vi "AsyncEngine.vi"(8 "Error In":errorcluster, 11 "AsyncDVR":refnum<data-value>) -> (0 "Error Out":errorcluster)   [LabVIEW 2019, in "MicronGRPCClient.lvclass"]
uses:
  MicronGRPCClient.lvclass
  Typedefs/AsyncCluster.ctl
  <vilib>/SLL Toolkit/SLL Queued State Machine/Queue Driver/Typedefs/Queue Type.ctl
  <vilib>/gRPC/LabVIEW gRPC Library/Shared/grpcId.ctl
  <vilib>/Utility/error.llb/DialogType.ctl
  <vilib>/SLL Toolkit/SLL Queued State Machine/Queue Driver/Enqueue an Item to Queue.vi
  <vilib>/SLL Toolkit/SLL Queued State Machine/Queue Driver/Dequeue Queue.vi
  <vilib>/SLL Toolkit/SLL Queued State Machine/Queue Driver/Enqueue N Items.vi
  <vilib>/SLL Toolkit/SLL Queued State Machine/Queue Driver/Flush Queue.vi
  <vilib>/SLL Toolkit/SLL Queued State Machine/Queue Driver/Release Queue.vi
  <vilib>/SLL Toolkit/SLL Queued State Machine/SLL QSM.lvlib
  <vilib>/gRPC/LabVIEW gRPC Library/grpc-lvsupport-release.lvlib
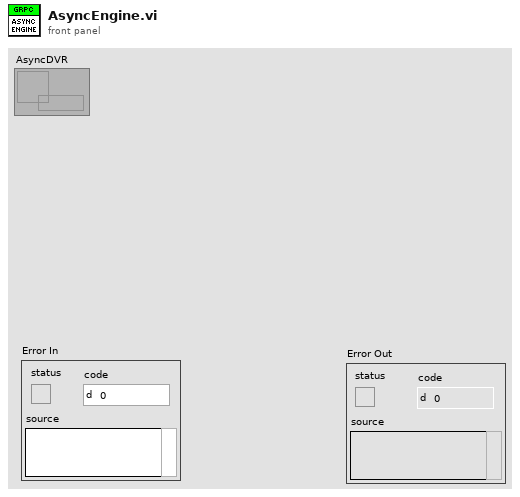
[diagram p1: front panel]
types:
  T1 = typedef "grpc-lvsupport-release.lvlib/grpcId.ctl" = u64
  T2 = cluster{"Flags":cluster{"Source Code?":bool}, "gRPC":cluster{"gRPC ID":T1, "PackageName":string, "ServiceName":string, "Simulate?":bool}}
  T3 = typedef "MicronGRPCClient.lvclass/AsyncCluster.ctl" = cluster{"QueueRef":refnum<queue>, "PackageName":string, "ServiceName":string, "gRPC ID":T1, "Simulate?":bool}
  T4 = typedef "DialogType.ctl" = u16
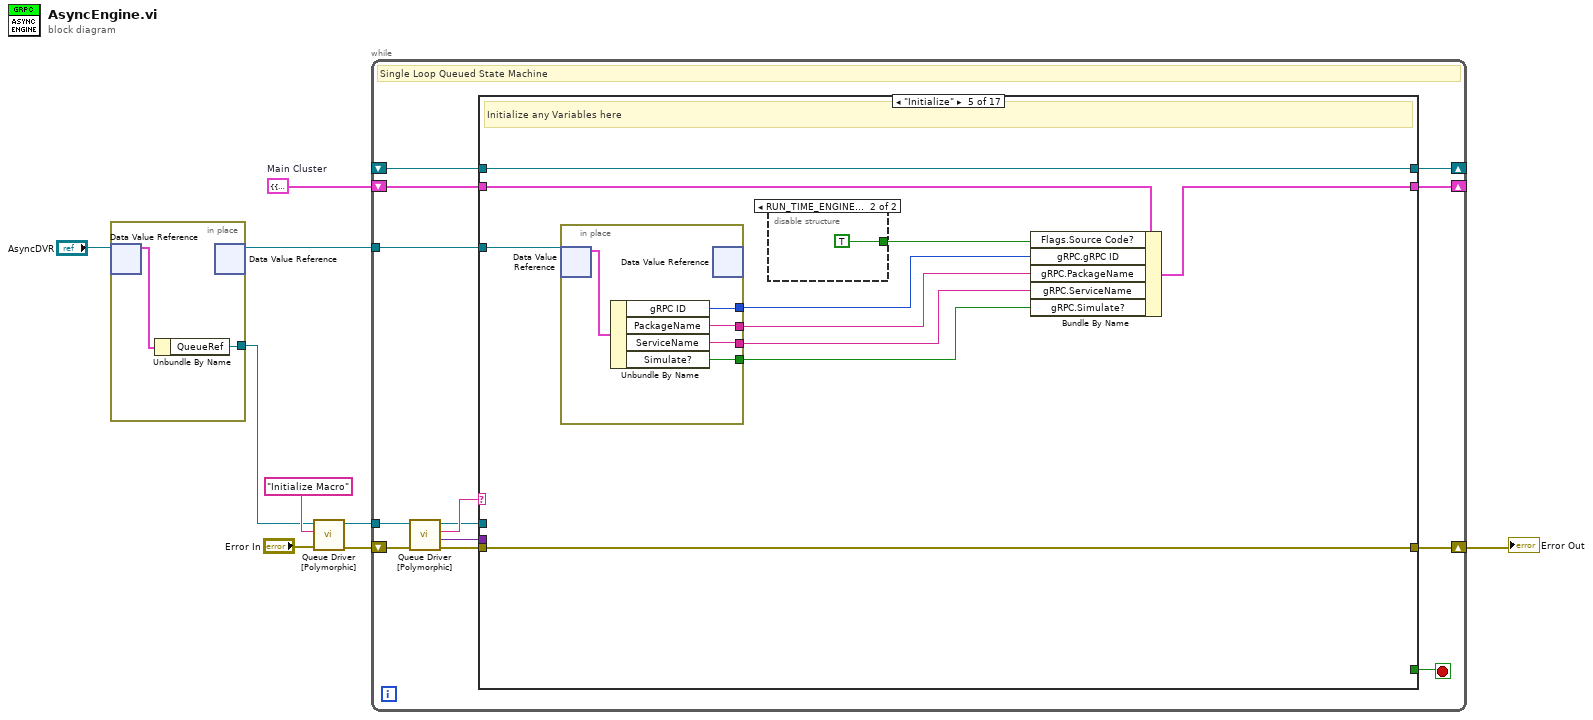
[diagram p0: block diagram]
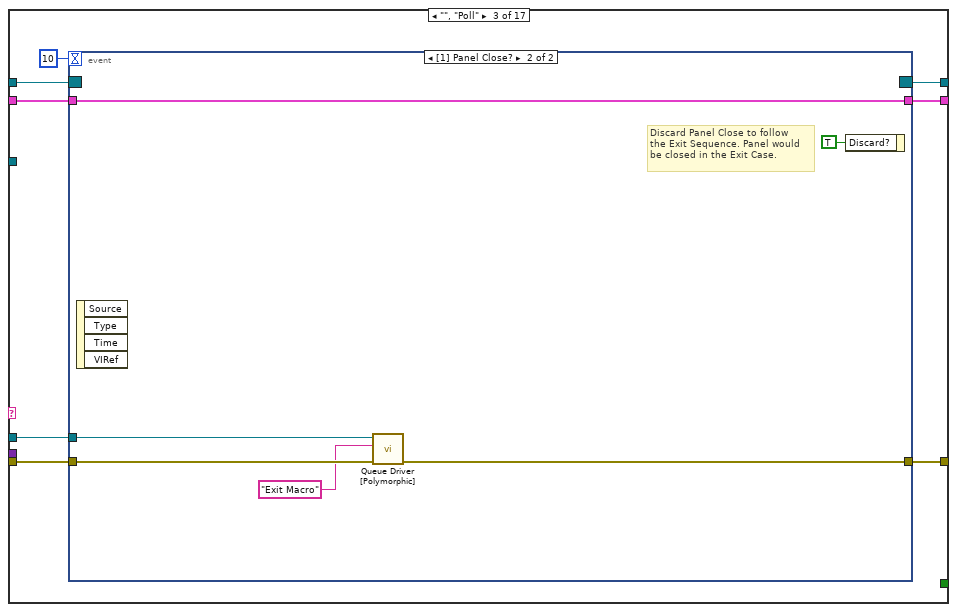
[diagram p4: hidden frame]
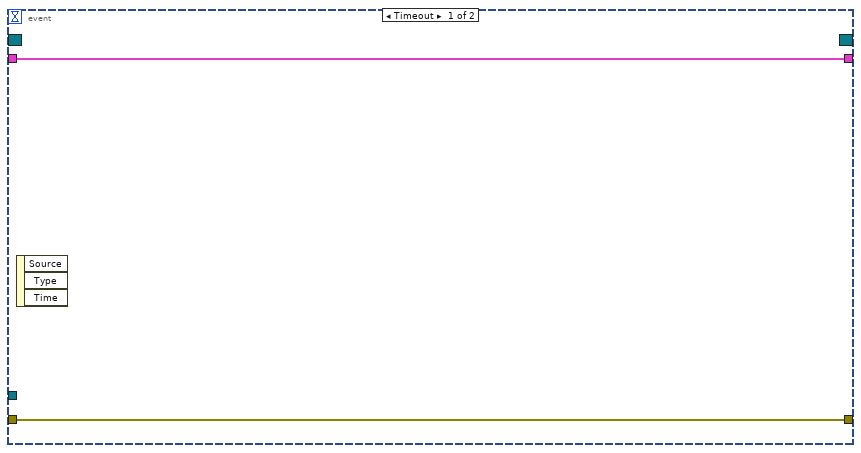
[diagram p5: hidden frame]
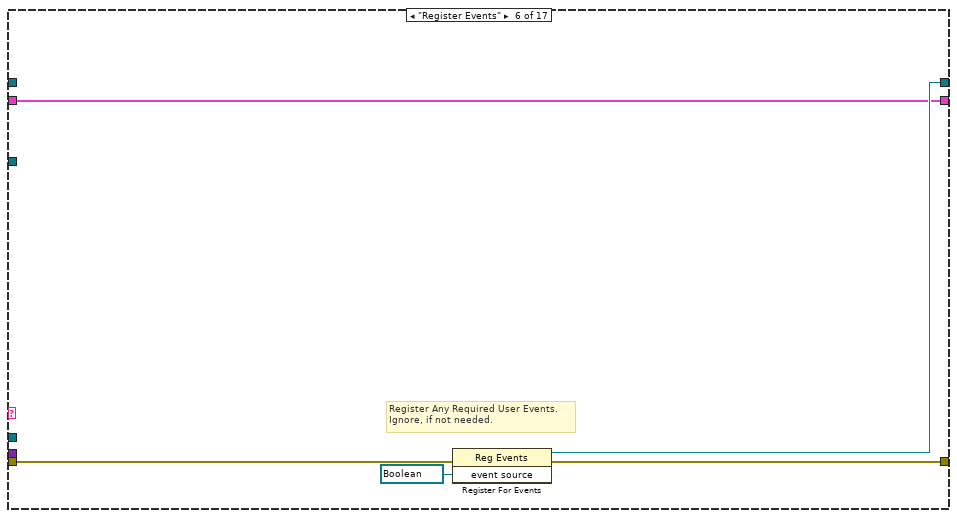
[diagram p8: hidden frame]
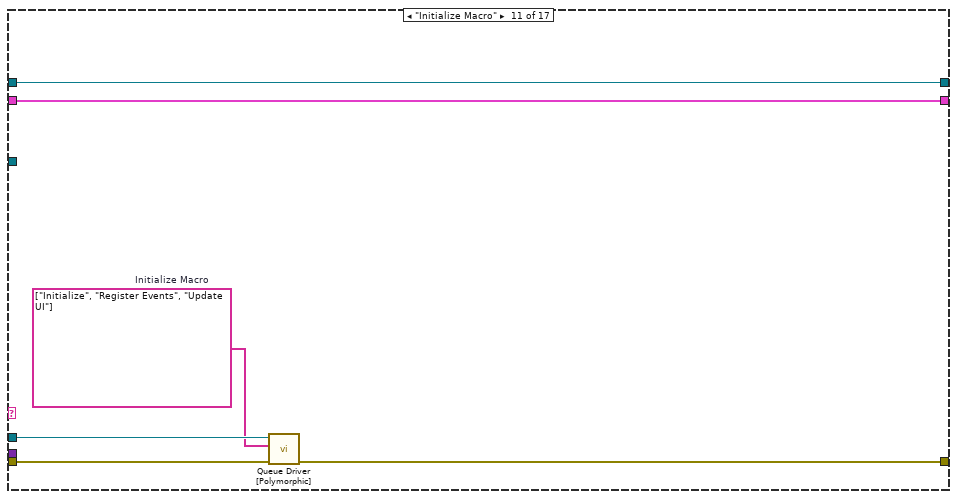
[diagram p13: hidden frame]
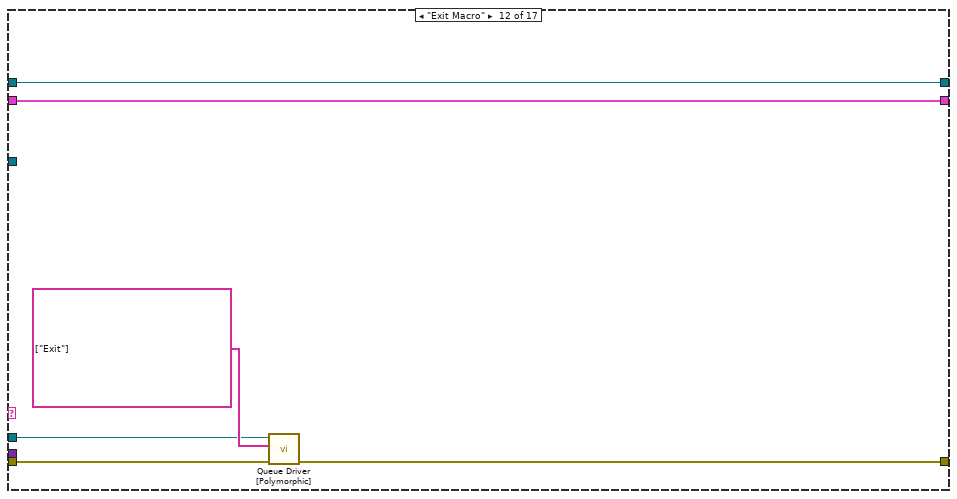
[diagram p14: hidden frame]
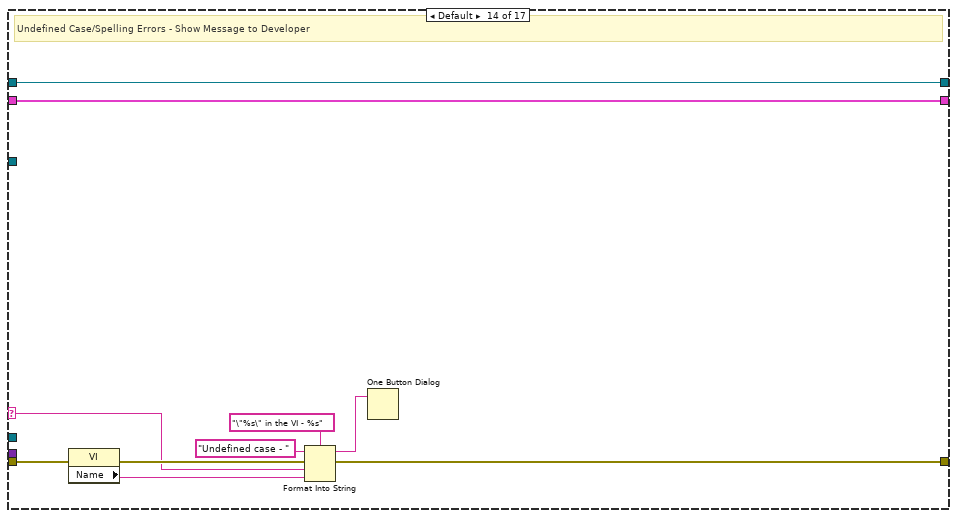
[diagram p16: hidden frame]
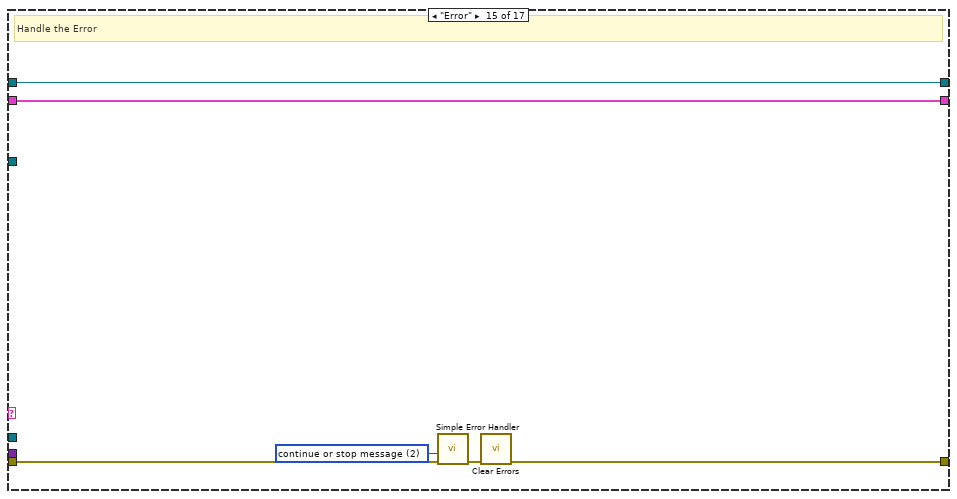
[diagram p17: hidden frame]
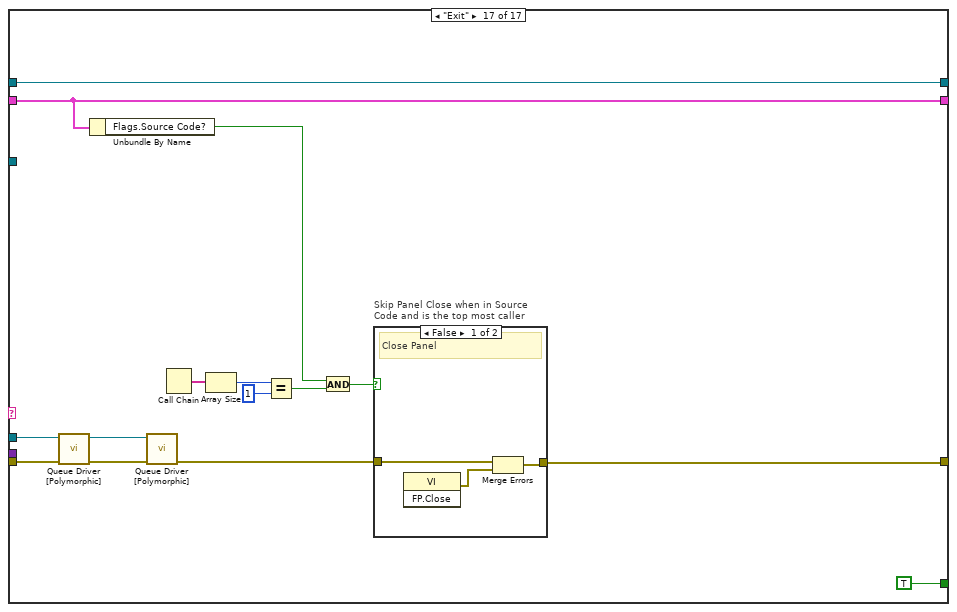
[diagram p19: hidden frame]
diagram:
  w7 = T2 {"Flags"={"Source Code?"=FALSE}, "gRPC"={"gRPC ID"=0, "PackageName"="", "ServiceName"="", "Simulate?"=FALSE}}  # Main Cluster
  n1 = in-place {
    in-place-border: [w10] -> w2
    n2 = in-place-dvr #1("AsyncDVR") -> (w11:T3)  [unwired: 1 out]
    n3 = Unbundle By Name(w11) -> ("QueueRef"=w10:refnum<queue>)
    n4 = in-place-dvr #1() -> (w1:refnum<data-value>)  [unwired: 1 in, 1 out]
  }
  n5 = call-poly <vilib>:"Queue Driver [Polymorphic].vi"("Error In"="Error In", "Item to Add"="Initialize Macro", "Queue Ref In"=w2) -> ("Error Out"=w6:errorcluster, "Queue Ref Out"=w9:refnum<queue>)  [unwired: 7 in]
  n6 = while "SLL Queued State Machine" {
    shift-right: [w22] -> w4
    shift-left: w6 -> [w24]
    shift-right: [w20] -> _
    shift-left: _ -> [w19]
    shift-right: [w18] -> _
    shift-left: w7 -> [w17]
    tunnel: w9 -> [w15]
    tunnel: w1 -> [w12]
    stop <- w21 stop-if-true
    # "Single Loop Queued State Machine"
    n7 = call-poly <vilib>:"Queue Driver [Polymorphic].vi"("Error In"=w24, "Queue Ref In"=w15) -> ("Error Out"=w23:errorcluster, "Data"=w13:variant, "Dequeue"=w16:string, "Queue Ref Out"=w14:refnum<queue>)  [unwired: 6 in]
    n8 = case "QSM Case Structure" shown="\"Initialize\"" w16 {
      selector: w16 -> [_ _ _ _ _ _ _ _ _ _ _ _ _ w98 _ _ _]
      tunnel: w23 -> [w27 w30 w36 w49 w59 w70 w73 w76 w79 w82 w86 w92 w97 w101 w113 w116 w129]
      tunnel: [w27 w30 w37 w49 w59 w69 w73 w76 w79 w82 w85 w91 w97 w104 w111 w116 w125] -> w22
      tunnel: [_ _ _ _ _ _ _ _ _ _ _ _ _ _ _ _ TRUE] -> w21
      tunnel: [w26 w29 w35 w48 w58 w68 w72 w75 w78 w81 w88 w94 w96 w107 w110 w115 w128] -> w20
      tunnel: w19 -> [w26 w29 w34 w48 w58 _ w72 w75 w78 w81 w88 w94 w96 w107 w110 w115 w128]
      tunnel: [w25 w28 w32 w47 w55 w67 w71 w74 w77 w80 w87 w93 w95 w106 w109 w114 w127] -> w18
      tunnel: w17 -> [w25 w28 w33 w47 w56 w67 w71 w74 w77 w80 w87 w93 w95 w106 w109 w114 w127]
      tunnel: w14 -> [_ _ w31 _ _ _ _ _ _ _ w84 w89 _ _ _ _ w118]
      tunnel: w13 -> [_ _ _ _ _ _ _ _ _ _ _ _ _ _ _ _ _]
      tunnel: w12 -> [_ _ _ _ w54 _ _ _ _ _ _ _ _ _ _ _ _]
      frame "/--------------- Read Me -----------------/" {
        # "General Purpose Queue Based State Machine for Any Use Case (main application, module, pop up message etc)\n\nAdvantages:\n1. Lean Project Code Base (dependencies are in vilib).\n2. This template can be safely used in multiple parallel running modules without any issues.\n3. This template can also be safely used even in cases where the VI is configured to be a clone, where multiple \ninstances of the VI could be executing concurrently.\n\nHow to Use:\n1. Add necessary items to the Main Cluster.\n2. Use the Polymorphic Queue Driver for doing any queue operations. \n3. Add any required user events in the \"Register Events\" case. Ignore if not needed.\n4. Use \"Macros\" section for defining any list of state calls, which could be used in multiple places. \nEx: Initialize Macro, might be needed if we need to any reinitialization."
      }
      frame "/------------------ Poll -------------------/" {
      }
      frame "", "Poll" {
        n9 = event shown="[1] Panel Close?" {
          selector: w34 -> [_ _]
          dyn-events: [_ _] -> w35
          timeout: 10 -> [_ _]
          tunnel: [w40 w45] -> w37
          tunnel: w36 -> [w40 w46]
          tunnel: w33 -> [w39 w44]
          tunnel: [w39 w44] -> w32
          tunnel: w31 -> [_ w42]
          event Timeout {
            n10 = event-data() -> ()  [unwired: 1 in, 3 out]
          }
          event Panel Close? {
            # "Discard Panel Close to follow\nthe Exit Sequence. Panel would\nbe closed in the Exit Case."
            n11 = event-data() -> ()  [unwired: 1 in, 4 out]
            n12 = call-poly <vilib>:"Queue Driver [Polymorphic].vi"("Error In"=w46, "Item to Add"="Exit Macro" ("Enqueue"), "Queue Ref In"=w42) -> ("Error Out"=w45:errorcluster)  [unwired: 7 in, 1 out]
            n13 = event-data("Discard?"=TRUE) -> ()  [unwired: 1 in, 1 out]
          }
        }
      }
      frame "/--------------- Initialize -----------------/" {
      }
      frame "Initialize" {
        # "Initialize any Variables here"
        n14 = in-place {
          in-place-border: [w63] -> w53
          in-place-border: [w62] -> w52
          in-place-border: [w61] -> w51
          in-place-border: [w60] -> w50
          n15 = in-place-dvr #2(w54) -> (w64:T3)  [unwired: 1 out]
          n16 = Unbundle By Name(w64) -> ("gRPC ID"=w63:T1, "PackageName"=w62:string, "ServiceName"=w61:string, "Simulate?"=w60:bool)
          n17 = in-place-dvr #2() -> ()  [unwired: 1 in, 2 out]
        }
        n18 = disable-structure shown="RUN_TIME_ENGINE==False" {
          disable-tunnel: [_ TRUE] -> w57
          frame condition #0 {
          }
          frame condition #1 (active) {
          }
        }
        n19 = Bundle By Name(cluster=w56, "Flags.Source Code?"=w57, "gRPC.gRPC ID"=w53, "gRPC.PackageName"=w52, "gRPC.ServiceName"=w51, "gRPC.Simulate?"=w50) -> (w55:T2)
      }
      frame "Register Events" {
        # "Register Any Required User Events. \nIgnore, if not needed."
        n20 = register-events(error in=w70, refnum<vi> refnum ("event source")) -> (reference out=w68:refnum<event-registration>, error out=w69:errorcluster)  [unwired: 1 in]
      }
      frame "/---------- Custom Case Splitter ----------/" {
      }
      frame "/-------------- User Interface --------------/" {
        # "Duplicate this case to create additional case splitters for readability"
      }
      frame "Update UI" {
        # "Update Front Panel Controls in this Case"
      }
      frame "/----------------- Macros -----------------/" {
      }
      frame "Initialize Macro" {
        w83 = string[] ["Initialize", "Register Events", "Update UI"]  # Initialize Macro
        n21 = call-poly <vilib>:"Queue Driver [Polymorphic].vi"("Error In"=w86, "Enqueue N"=w83, "Queue Ref In"=w84) -> ("Error Out"=w85:errorcluster)  [unwired: 7 in, 1 out]
      }
      frame "Exit Macro" {
        n22 = call-poly <vilib>:"Queue Driver [Polymorphic].vi"("Error In"=w92, "Enqueue N"=string[] ["Exit"], "Queue Ref In"=w89) -> ("Error Out"=w91:errorcluster)  [unwired: 7 in, 1 out]
      }
      frame "/-------------- Error Handler--------------/" {
      }
      frame Default {
        # "Undefined Case/Spelling Errors - Show Message to Developer"
        n23 = property class="VI"(error in=w101) -> (error out=w100:errorcluster, "Name"=w99:string)  [unwired: 1 in, 1 out]
        n24 = Format Into String(format string="\"%s\" in the VI - %s" ("message"), initial string="Undefined case - ", error in=w100, w98, w99) -> (resulting string=w102:string, error out=w104:errorcluster)
        n25 = One Button Dialog(message=w102) -> ()  [unwired: 1 in, 1 out]
      }
      frame "Error" {
        w108 = T4 2 items=["no dialog", "OK message", "continue or stop message", "OK message + warnings", "continue/stop + warnings"] ("type of dialog (OK msg:1)")
        # "Handle the Error"
        n26 = call <vilib>:"Simple Error Handler.vi"("type of dialog (OK msg:1)"=w108, "error in (no error)"=w113) -> ("error out"=w112:errorcluster)  [unwired: 3 in, 4 out]
        n27 = call <vilib>:"Clear Errors.vi"("error in (no error)"=w112) -> ("error out"=w111:errorcluster)  [unwired: 5 in, 1 out]
      }
      frame "/------------------- Exit --------------------/" {
      }
      frame "Exit" {
        n28 = call-poly <vilib>:"Queue Driver [Polymorphic].vi"("Error In"=w129, "Queue Ref In"=w118) -> ("Error Out"=w130:errorcluster, "Queue Ref Out"=w117:refnum<queue>)  [unwired: 7 in, 1 out]
        n29 = Unbundle By Name(w127) -> ("Flags.Source Code?"=w120:bool)
        n30 = call-poly <vilib>:"Queue Driver [Polymorphic].vi"("Error In"=w130, "Queue Ref In"=w117) -> ("Error Out"=w126:errorcluster)  [unwired: 9 in]
        n31 = Call Chain() -> (call chain=w124:string[])
        n32 = Array Size(array=w124) -> (size(s)=w123:i32)
        n33 = Equal?(x=w123, y=1) -> (x = y?=w121:bool)
        n34 = And(x=w120, y=w121) -> (x .and. y?=w119:bool)
        n35 = case "Skip Panel Close when in Source\nCode and is the top most caller" shown="False" w119 {
          tunnel: w126 -> [w133 w135]
          tunnel: [w134 w135] -> w125
          frame False {
            # "Close Panel"
            n36 = invoke class="VI" method="FP.Close"() -> (error out=w132:errorcluster)  [unwired: 3 in, 2 out]
            n37 = Merge Errors(w133, w132) -> (w134:errorcluster)
          }
          frame True {
            # "Do Not Close Panel"
          }
        }
      }
    }
  }
  "Error Out" <- w4
